vi "AdaptToInputs.vi"(3 "Term Types":T1[](array[typedef]), 4 "XRef":refnum<vi>, 5 "State In":T4) -> (0 "Reply":string[](array[string]), 2 "State Out":T4)   [LabVIEW 2017]
uses:
  <vilib>/UPVI/lvhdf5/xnodehelpers/State.ctl
  <vilib>/UPVI/lvhdf5/xnodehelpers/TermsPlus.ctl
  <vilib>/XNodeSupport/XNodeTerm3.ctl
  <vilib>/XNodeSupport/XNodeString.ctl
  <vilib>/XNodeSupport/XNodeVariant.ctl
  <vilib>/XNodeSupport/XNodeRect32.ctl
  <vilib>/XNodeSupport/XNodeInt.ctl
  <vilib>/XNodeSupport/XNodeBool.ctl
  <vilib>/XNodeSupport/XNodeTermDirection.ctl
  <vilib>/UPVI/lvhdf5/xnodehelpers/TermBehavior.ctl
  <vilib>/XNodeSupport/XNodeError3Array.ctl
  <vilib>/XNodeSupport/XNodeError3.ctl
  <vilib>/XNodeSupport/XNodeTermTypeIDPair.ctl
  <vilib>/XNodeSupport/XNodeType.ctl
  <vilib>/Utility/VariantDataType/Type.ctl
  <vilib>/Utility/error.llb/DialogType.ctl
  <vilib>/Utility/VariantDataType/VariantType.lvlib
  <vilib>/XNodeSupport/NI_XNodeSupport.lvlib
panel:
  # "LVHDF5 Toolkit\nCopyright (c) 2005-2013 by Jason D. Sommerville\nCopyright (c) 2014 by UPVI, LLC.\n\nThis use and distribution of this file is governed by the terms found in \nLICENSE.txt distributed with this toolkit and installed at\n <user.lib>\\_lvhdf5\\LICENSE.txt"
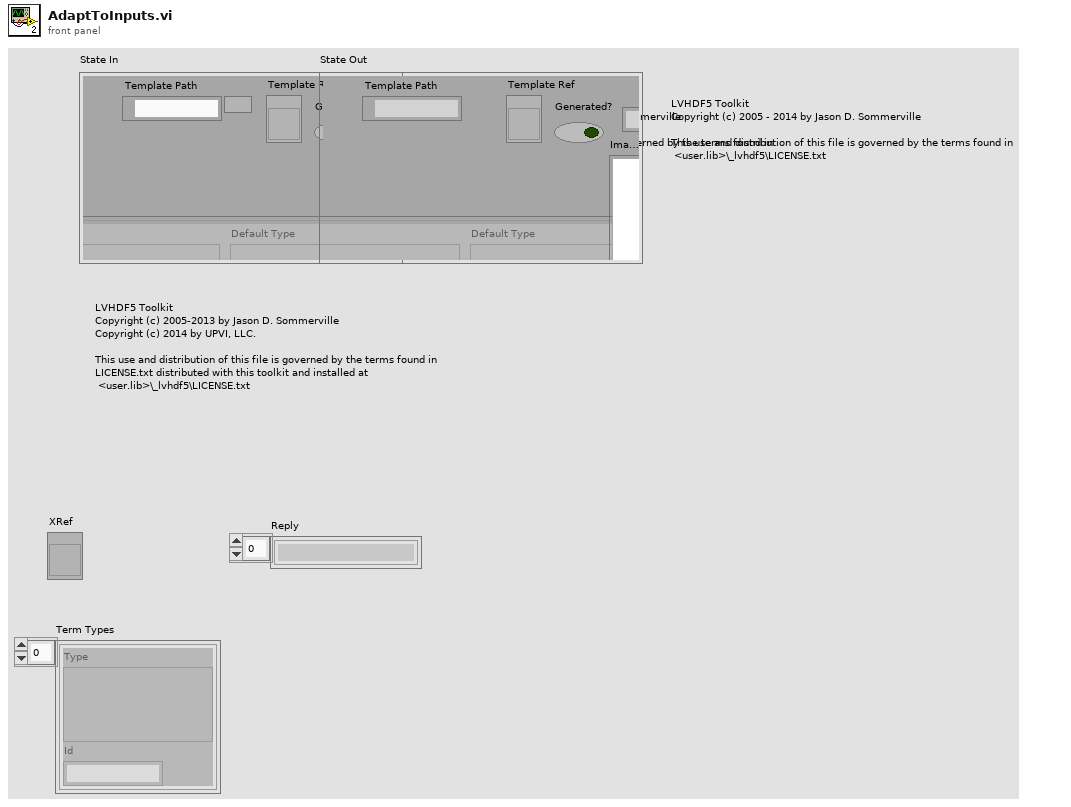
[diagram p1: front panel]
types:
  T1 = typedef "NI_XNodeSupport.lvlib/XNodeTermTypeIDPair.ctl" = cluster{"Type":T2, "Id":T3}
  T2 = typedef "NI_XNodeSupport.lvlib/XNodeType.ctl" = variant
  T3 = typedef "NI_XNodeSupport.lvlib/XNodeString.ctl" = string
  T4 = typedef "State.ctl" = cluster{"Template Path":path, "Template Ref":refnum<vi>, "Terms":T5[], "Display Name":string, "Image":picture, "Errors":T13, "Generated?":bool}
  T5 = typedef "TermsPlus.ctl" = cluster{"Term 3":T6, "Default Type":variant, "Behavior":T12, "Behavior Arg":string, "WiredResponse":bool, "Wired":enum16{"Unknown", "Unwired", "Wired"}}
  T6 = typedef "NI_XNodeSupport.lvlib/XNodeTerm3.ctl" = cluster{"Name":T3, "Id":T3, "Type":T7, "Bounds":T8, "Input?":T10, "Required?":T10, "Recommended?":T10, "Adaptive?":T10, "Hidden?":T10, "Direction":T11, "Break Wire?":T10}
  T7 = typedef "NI_XNodeSupport.lvlib/XNodeVariant.ctl" = variant
  T8 = typedef "NI_XNodeSupport.lvlib/XNodeRect32.ctl" = cluster{"Left":T9, "Top":T9, "Right":T9, "Bottom":T9}
  T9 = typedef "NI_XNodeSupport.lvlib/XNodeInt.ctl" = i32
  T10 = typedef "NI_XNodeSupport.lvlib/XNodeBool.ctl" = bool
  T11 = typedef "NI_XNodeSupport.lvlib/XNodeTermDirection.ctl" = enum32{"Auto", "Up", "Down", "Left", "Right", "Center"}
  T12 = typedef "TermBehavior.ctl" = enum16{"Normal", "Anything", "LVType", "Path or Ref", "Attr Name", "Attr Poly", "Elt Poly", "Dset Poly", "WDT Poly"}
  T13 = typedef "NI_XNodeSupport.lvlib/XNodeError3Array.ctl" = T14[]
  T14 = typedef "NI_XNodeSupport.lvlib/XNodeError3.ctl" = cluster{"Error":T3, "Details":T3, "Help File":T3, "Help Topic":T3}
  T15 = typedef "VariantType.lvlib/Type.ctl" = enum8{"Invalid Type", "Void", "I8", "I16", "I32", "I64", "U8", "U16", "U32", "U64", "Single Float", "Double Float", "Extended Float", "Single Complex", "Double Complex", "Extended Complex", "Enum U8", "Enum U16", "Enum U32", "Enum U64", "Single Float With Unit", "Double Float With Unit", "Extended Float With Unit", "Single Complex with Unit", "Double Complex with Unit", "Extended Complex with Unit", "Boolean", "String", "Path", "Picture", "Tag", "Array", "Cluster", "Variant", "LV Variant", "Waveform", "Timestamp", "Digital Waveform", "Digital Data", "ExpressData", "Refnum", "External Data", "VI", "Poly VI", "LabVIEW Class Instance", "Fixed Point"}
  T16 = typedef "HDF5 Ref.ctl" = refnum<k1>
  T17 = typedef "DialogType.ctl" = u16
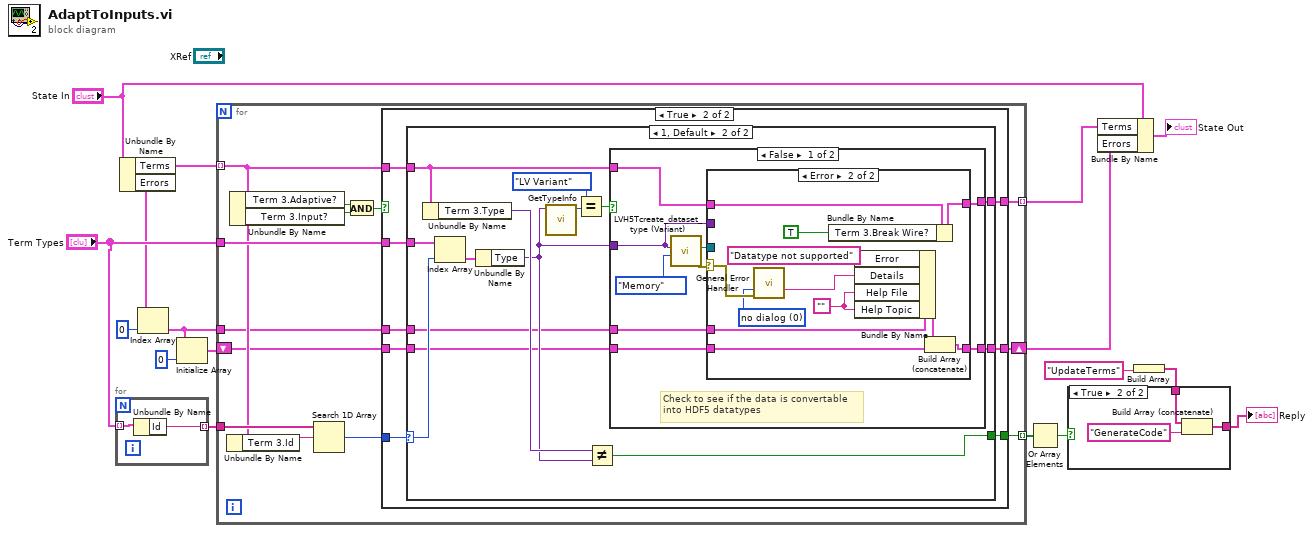
[diagram p0: block diagram]
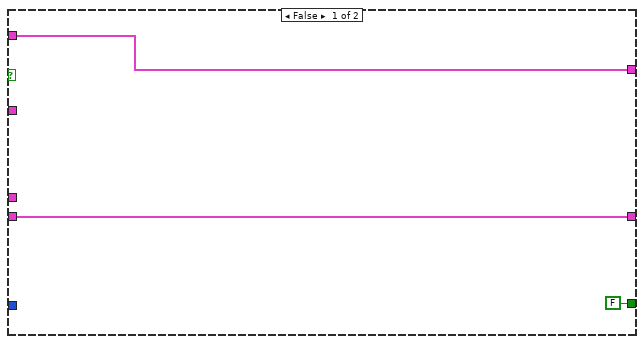
[diagram p3: hidden frame]
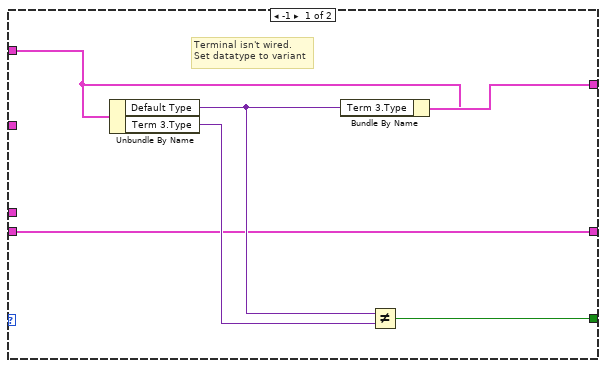
[diagram p4: hidden frame]
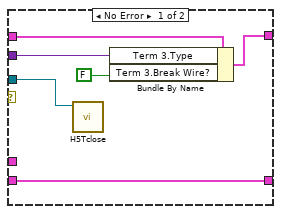
[diagram p5: hidden frame]
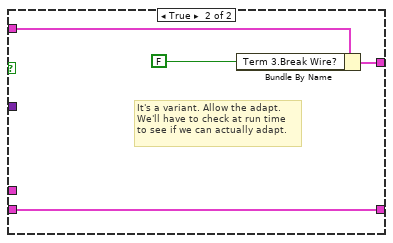
[diagram p6: hidden frame]
diagram:
  n1 = for {
    tunnel: [w19] -> w14 mode=indexing
    tunnel: "Term Types" -> [w18] mode=indexing
    n2 = Unbundle By Name(w18) -> ("Id"=w19:T3)
  }
  n3 = Unbundle By Name("State In") -> ("Terms"=w16:T5[], "Errors"=w10:T13)
  n4 = Index Array(array=w10, index=0) -> (element=w6:T14)
  n5 = Initialize Array(w6, 0 ("dimension size")) -> (w7:T14[])
  n6 = for {
    tunnel: w16 -> [w27] mode=indexing
    tunnel: w14 -> [w32]
    tunnel: "Term Types" -> [w30]
    tunnel: [w29] -> w13 mode=indexing
    tunnel: [w26] -> w12 mode=indexing
    shift-right: [w23] -> w8
    shift-left: w7 -> [w25]
    tunnel: w6 -> [w24]
    n7 = Unbundle By Name(w27) -> ("Term 3.Id"=w31:T3)
    n8 = Unbundle By Name(w27) -> ("Term 3.Adaptive?"=w22:T10, "Term 3.Input?"=w21:T10)
    n9 = Search 1D Array(1D array=w32, element=w31) -> (index of element=w28:i32)  [unwired: 1 in]
    n10 = And(x=w22, y=w21) -> (x .and. y?=w20:T10)
    n11 = case shown="True" w20 {
      tunnel: w30 -> [_ w43]
      tunnel: w27 -> [w35 w42]
      tunnel: [w35 w41] -> w29
      tunnel: w28 -> [_ w40]
      tunnel: [FALSE w39] -> w26
      tunnel: w25 -> [w33 w38]
      tunnel: w24 -> [_ w37]
      tunnel: [w33 w36] -> w23
      frame False {
      }
      frame True {
        n12 = case shown="1, Default" w40 {
          selector: w40 -> [_ w57]
          tunnel: w43 -> [_ w61]
          tunnel: w42 -> [w48 w56]
          tunnel: [w49 w59] -> w41
          tunnel: [w45 w53] -> w39
          tunnel: w38 -> [w44 w52]
          tunnel: w37 -> [_ w51]
          tunnel: [w44 w50] -> w36
          frame -1 {
            # "Terminal isn't wired.\nSet datatype to variant"
            n13 = Unbundle By Name(w48) -> ("Default Type"=w47:variant, "Term 3.Type"=w46:T7)
            n14 = Bundle By Name(cluster=w48, "Term 3.Type"=w47) -> (w49:T5)
            n15 = Not Equal?(x=w47, y=w46) -> (x != y?=w45:bool)
          }
          frame 1, Default {
            n16 = Unbundle By Name(w56) -> ("Term 3.Type"=w55:T7)
            n17 = Index Array(array=w61, index=w57) -> (element=w60:T1)
            n18 = Unbundle By Name(w60) -> ("Type"=w54:T2)
            n19 = call <vilib>:"GetTypeInfo.vi"("Variant"=w54) -> ("Type Enum"=w62:T15)  [unwired: 6 in, 4 out]
            n20 = Equal?(x=Type."LV Variant" ("Type Enum"), y=w62) -> (x = y?=w58:bool)
            n21 = Not Equal?(x=w55, y=w54) -> (x != y?=w53:bool)
            n22 = case shown="False" w58 {
              tunnel: w56 -> [w69 w94]
              tunnel: [w67 w92] -> w59
              tunnel: w54 -> [w68 _]
              tunnel: w52 -> [w66 w91]
              tunnel: w51 -> [w65 _]
              tunnel: [w64 w91] -> w50
              frame False {
                # "Check to see if the data is convertable\ninto HDF5 datatypes"
                n23 = call <vilib>:"LVH5Tcreate_dataset_type (Variant).vi"("Type"=enum16{"File", "Memory"}."Memory", "Data"=w68) -> ("error out"=w71:errorcluster, "HDF5 Type Ref"=w70:T16)  [unwired: 5 in, 3 out]
                n24 = case shown="Error" w71 {
                  selector: w71 -> [_ w86]
                  tunnel: w70 -> [w78 _]
                  tunnel: w69 -> [w77 w90]
                  tunnel: w68 -> [w75 _]
                  tunnel: [w74 w88] -> w67
                  tunnel: w66 -> [w73 w81]
                  tunnel: w65 -> [_ w87]
                  tunnel: [w73 w79] -> w64
                  frame No Error {
                    n25 = call <vilib>:"H5Tclose.vi"("HDF5 Datatype Ref"=w78) -> ()  [unwired: 8 in, 1 out]
                    n26 = Bundle By Name(cluster=w77, "Term 3.Type"=w75, "Term 3.Break Wire?"=FALSE ("Broken")) -> (w74:T5)
                  }
                  frame Error {
                    w82 = ""
                    w85 = T17 0 items=["no dialog", "OK message", "continue or stop message", "OK message + warnings", "continue/stop + warnings"] ("type of dialog (OK msg:1)")
                    n27 = call <vilib>:"General Error Handler.vi"("type of dialog (OK msg:1)"=w85, "error in (no error)"=w86) -> ("message"=w84:string)  [unwired: 9 in, 4 out]
                    n28 = Bundle By Name(cluster=w90, "Term 3.Break Wire?"=TRUE ("Broken")) -> (w88:T5)
                    n29 = Bundle By Name(cluster=w87, "Error"=T3 "Datatype not supported", "Details"=w84, "Help File"=w82, "Help Topic"=w82) -> (w80:T14)
                    n30 = Build Array (concatenate)(w80, w81) -> (w79:T14[])
                  }
                }
              }
              frame True {
                # "It's a variant. Allow the adapt.\nWe'll have to check at run time\nto see if we can actually adapt."
                n31 = Bundle By Name(cluster=w94, "Term 3.Break Wire?"=FALSE ("Broken")) -> (w92:T5)
              }
            }
          }
        }
      }
    }
  }
  n32 = Or Array Elements(Boolean array=w12) -> (logical OR=w2:bool)
  n33 = Bundle By Name(cluster="State In", "Terms"=w13, "Errors"=w8) -> (→"State Out":T4)
  n34 = Build Array("UpdateTerms" ("String")) -> (w3:string[])
  n35 = case shown="True" w2 {
    tunnel: w3 -> [w95 w97]
    tunnel: [w95 w96] -> w1
    frame False {
    }
    frame True {
      n36 = Build Array (concatenate)(w97, "GenerateCode" ("String")) -> (w96:string[])
    }
  }
  "Reply" <- w1
